vi "GIF.Read.Unpack__ogtk.vi"(6 "error in (no error)":errorcluster, 9 "Raw GIF89a bytes":u8[](array[numeric]) format="%.0x") -> (0 "error out":errorcluster, 2 "Delay (ms)":u32[](array[numeric]), 3 "Picture Array":T1[](array[typedef]))   [LabVIEW 2011]
uses:
  <vilib>/picture/picture.llb/imagedata.ctl
panel:
  out "Unpack in-progress":T2
  # "GIF.Read.Unpack.vi\n\nUnpacks image(s) from a raw GIF format.\n\nPlease visit http://www.OpenG.org to learn about the\nOpen Source LabVIEW software movement.\n\nNOTICE -- YOU MUST LEAVE THIS NOTICE IN PLACE.  PER THE TERMS OF THE LICENSE BELOW, YOU MAY SUBLICENSE THIS SOFTWARE \nIN ANY WAY THAT DOES NOT CONFLICT WITH THIS LICENSE.\n\n### BSD License (http://www.opensource.org/licenses/bsd-license.php) Begin ###\n \nCopyright (c) 2007, Bill Clench <bclench@yahoo.com>\n\nAll rights reserved.\n\nRedistribution and use in source and binary forms, with or without modification, are permitted provided that the following conditions are met:\n\n    * Redistributions of source code must retain the above copyright notice, this list of conditions and the following disclaimer.\n    * Redistributions in binary form must reproduce the above copyright notice, this list of conditions and the following disclaimer in the \n       documentation and/or other materials provided with the distribution.\n    * Neither the name of SciWare, James Kring, Inc., nor the names of its contributors may be used to endorse or promote products derived \n       from this software without specific prior written permission.\n\nTHIS SOFTWARE IS PROVIDED BY THE COPYRIGHT HOLDERS AND CONTRIBUTORS \"AS IS\" AND ANY EXPRESS OR IMPLIED WARRANTIES, \nINCLUDING, BUT NOT LIMITED TO, THE IMPLIED WARRANTIES OF MERCHANTABILITY AND FITNESS FOR A PARTICULAR PURPOSE ARE \nDISCLAIMED. IN NO EVENT SHALL THE COPYRIGHT OWNER OR CONTRIBUTORS BE LIABLE FOR ANY DIRECT, INDIRECT, INCIDENTAL,\n SPECIAL, EXEMPLARY, OR CONSEQUENTIAL DAMAGES (INCLUDING, BUT NOT LIMITED TO, PROCUREMENT OF SUBSTITUTE GOODS OR \nSERVICES; LOSS OF USE, DATA, OR PROFITS; OR BUSINESS INTERRUPTION) HOWEVER CAUSED AND ON ANY THEORY OF LIABILITY, \nWHETHER IN CONTRACT, STRICT LIABILITY, OR TORT (INCLUDING NEGLIGENCE OR OTHERWISE) ARISING IN ANY WAY OUT OF THE USE \nOF THIS SOFTWARE, EVEN IF ADVISED OF THE POSSIBILITY OF SUCH DAMAGE.\n\n### BSD License End ###"
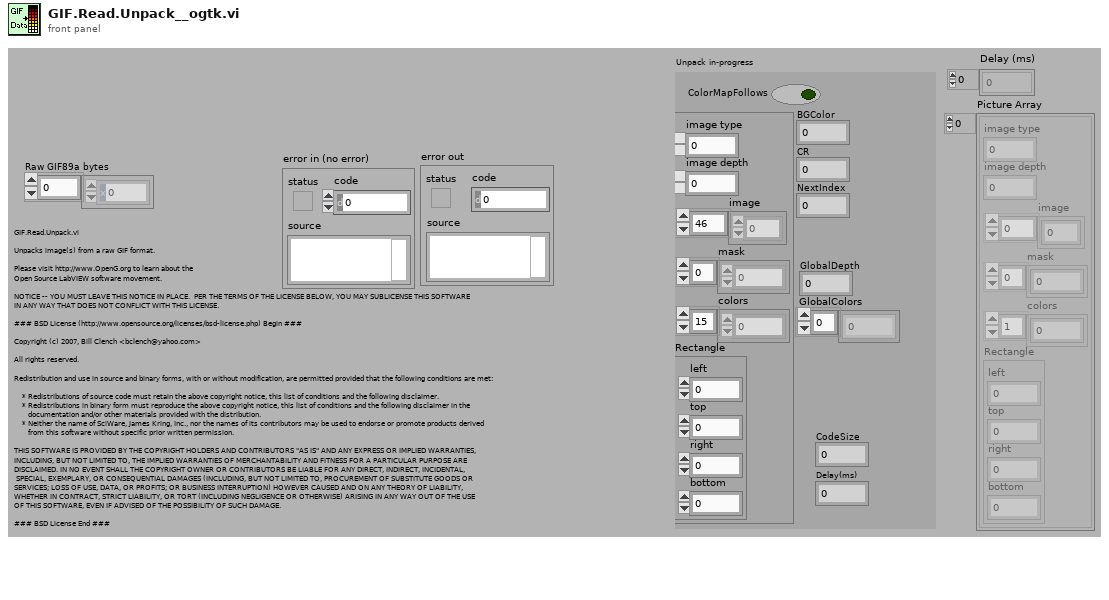
[diagram p1: front panel]
types:
  T1 = typedef "imagedata.ctl" = cluster{"image type":i32, "image depth":i32, "image":u8[], "mask":u8[], "colors":u32[], "Rectangle":cluster{"left":i16, "top":i16, "right":i16, "bottom":i16}}
  T2 = cluster{"ColorMapFollows":bool, "image data":T1, "BGColor":u8, "CR":u8, "NextIndex":i32, "GlobalDepth":i32, "CodeSize":i32, "Delay(ms)":i32, "GlobalColors":u32[]}
  T3 = enum16{"Begin", "Header", "LS_LSDescriptor", "LS_GCTable", "Data_LGD_SPB", "Data_GB_GRB_PTE", "Data_GB_GCE", "Data_GB_GRB_TBI_IDesc", "Data_GB_GRB_TBI_CMap", "Data_GB_GRB_TBI_ImageData", "End_Of_File"}
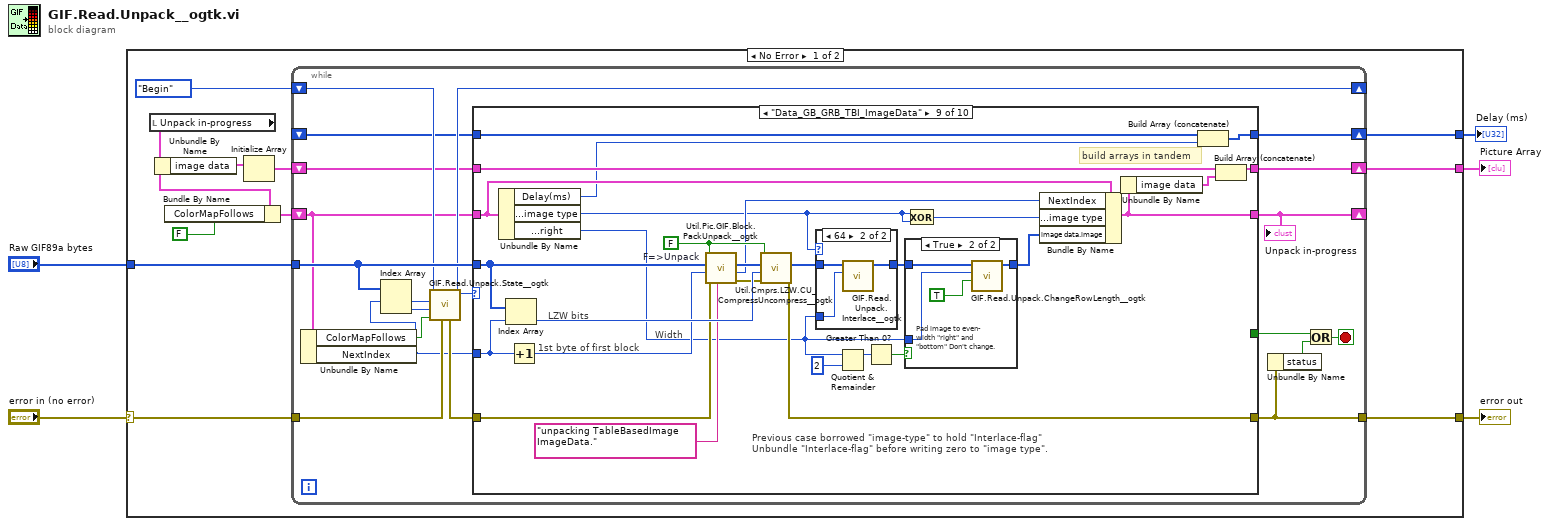
[diagram p0: block diagram]
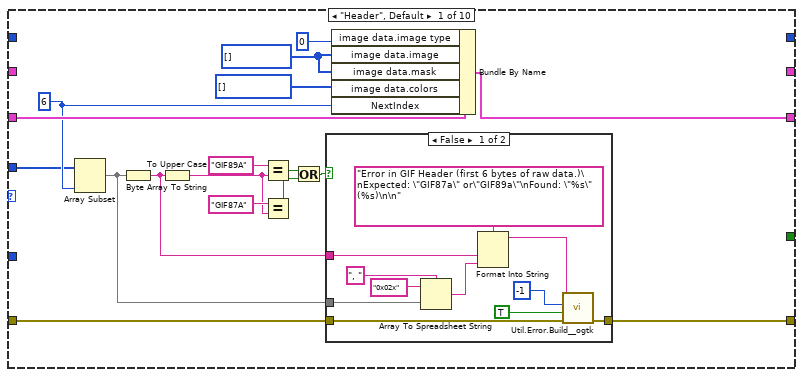
[diagram p2: hidden frame]
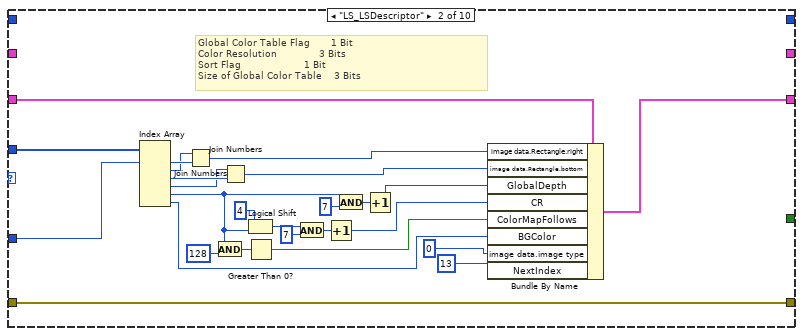
[diagram p4: hidden frame]
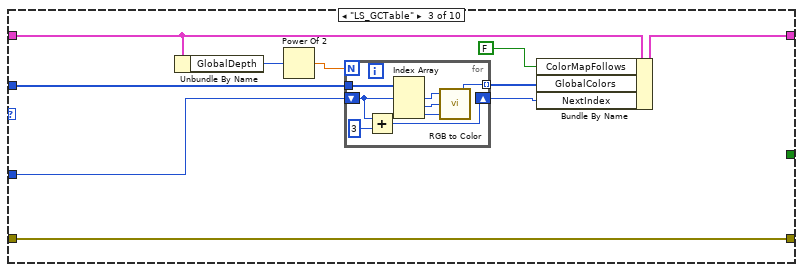
[diagram p5: hidden frame]
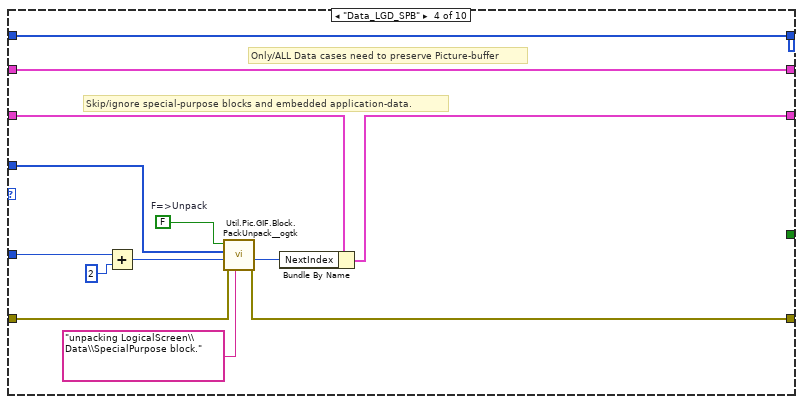
[diagram p6: hidden frame]
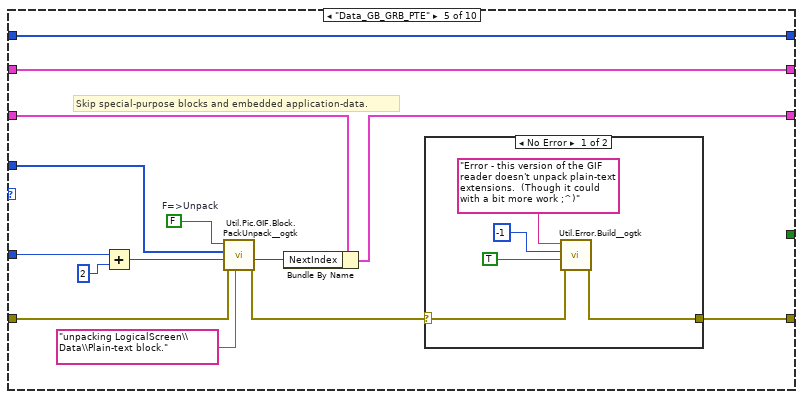
[diagram p7: hidden frame]
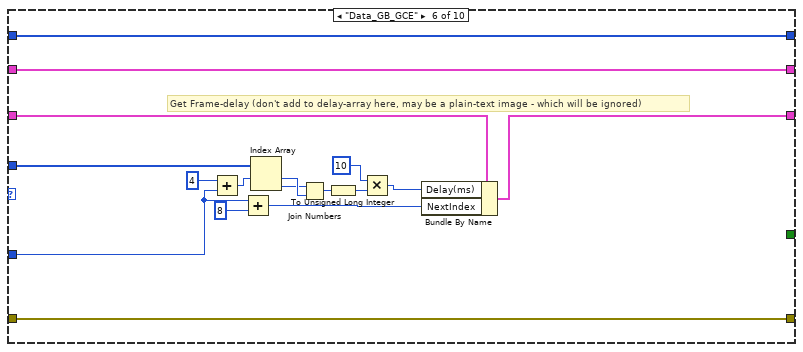
[diagram p9: hidden frame]
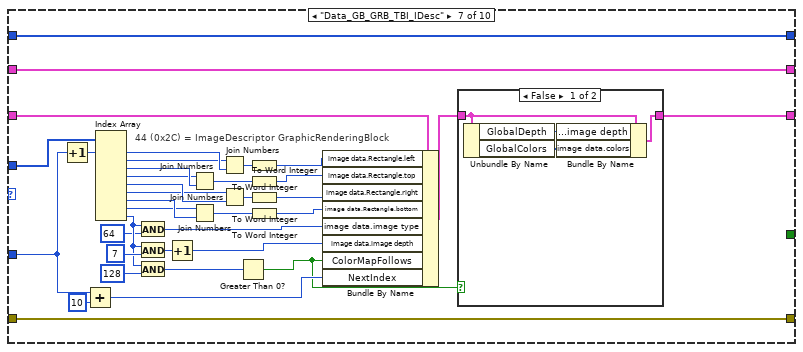
[diagram p10: hidden frame]
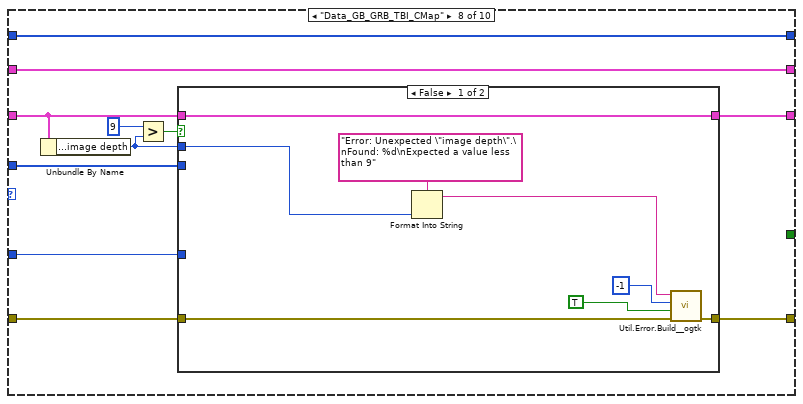
[diagram p12: hidden frame]
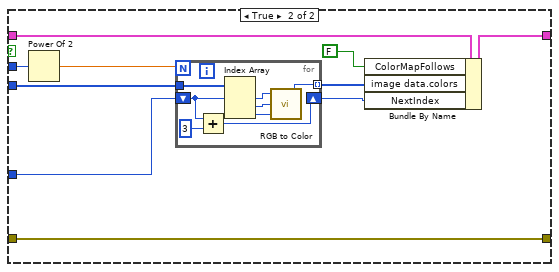
[diagram p13: hidden frame]
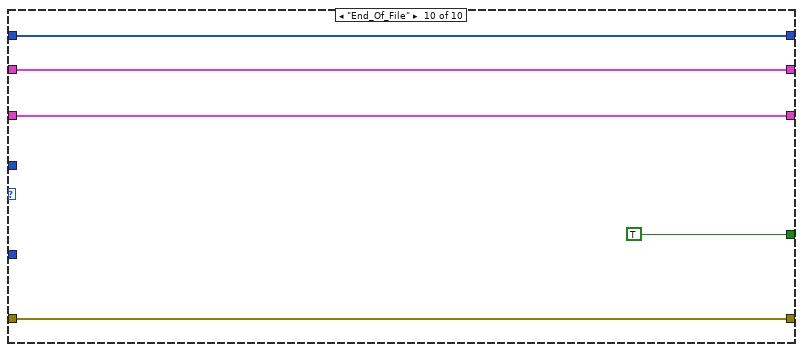
[diagram p16: hidden frame]
diagram:
  n1 = case shown="No Error" "error in (no error)" {
    selector: "error in (no error)" -> [w12 w279]
    tunnel: "Raw GIF89a bytes" -> [w16 _]
    tunnel: [w15 w279] -> w4
    tunnel: [w7 _] -> w2
    tunnel: [w6 _] -> w1
    frame No Error {
      n2 = local read "Unpack in-progress"() -> (w11:T2)
      n3 = Unbundle By Name(w11) -> ("image data"=w10:T1)
      n4 = Bundle By Name(cluster=w11, "ColorMapFollows"=FALSE) -> (w14:T2)
      n5 = Initialize Array(w10) -> (w9:T1[])  [unwired: 1 in]
      n6 = while {
        shift-right: [w28] -> _
        shift-left: w14 -> [w23]
        shift-right: [w26] -> _
        shift-left: T3."Begin" -> [w27]
        tunnel: w16 -> [w35]
        tunnel: [w32] -> w15
        tunnel: w12 -> [w25]
        shift-right: [w21] -> w7
        shift-left: w9 -> [w22]
        shift-right: [w18] -> w6
        shift-left: _ -> [w17]
        stop <- w30 stop-if-true
        n7 = Unbundle By Name(w23) -> ("ColorMapFollows"=w20:bool, "NextIndex"=w19:i32)
        n8 = Index Array(array=w35, index #1=w19) -> (element #1=w34:u8, element #2=w33:u8)  [unwired: 1 in]
        n9 = call "GIF.Read.Unpack.State__ogtk.vi"("error in (no error)"=w25, "ColorMap"=w20, "NextLabel"=w33, "NextCharacter"=w34, "State in"=w27) -> ("New State"=w26:T3, "error out"=w24:errorcluster)  [unwired: 5 in]
        n10 = case shown="\"Data_GB_GRB_TBI_ImageData\"" w26 {
          tunnel: w23 -> [w52 w68 w94 w120 w134 w150 w168 w208 w253 w278]
          tunnel: [w41 w65 w96 w119 w133 w149 w165 w207 w242 w278] -> w28
          tunnel: w35 -> [w40 w71 w98 w115 w129 w151 w171 w209 w260 _]
          tunnel: [w39 w66 w92 w112 w123 w147 w164 w201 w259 w276] -> w32
          tunnel: w19 -> [_ w67 w97 w118 w132 w148 w163 w210 w237 _]
          tunnel: [_ _ _ _ _ _ _ _ _ TRUE] -> w29
          tunnel: w24 -> [w37 w66 w92 w113 w126 w147 w164 w202 w249 w276]
          tunnel: w22 -> [_ _ _ w117 w131 w146 w170 w206 w257 w275]
          tunnel: [_ _ _ w117 w131 w146 w170 w206 w256 w275] -> w21
          tunnel: w17 -> [_ _ _ w109 w122 w142 w159 w200 w240 w274]
          tunnel: [_ _ _ w109 w122 w142 w159 w200 w239 w274] -> w18
          frame "Header", Default {
            w51 = u8[] []
            w42 = 6
            n11 = Array Subset(array=w40, length=w42) -> (w38:u8[])  [unwired: 1 in]
            n12 = Byte Array To String(unsigned byte array=w38) -> (string=w36:string)
            n13 = To Upper Case(1:w36) -> (0:w43:string)
            n14 = Equal?(x="GIF89A", y=w43) -> (x = y?=w47:bool)
            n15 = Equal?(x="GIF87A", y=w43) -> (x = y?=w46:bool)
            n16 = Or(x=w47, y=w46) -> (x .or. y?=w45:bool)
            n17 = case shown="False" w45 {
              tunnel: [w61 w64] -> w39
              tunnel: w36 -> [w62 _]
              tunnel: w38 -> [w57 _]
              tunnel: w37 -> [w53 w64]
              frame False {
                n18 = Array To Spreadsheet String(delimiter (Tab)=", ", array=w57, 3:"0x02x") -> (spreadsheet string=w54:string)
                n19 = Format Into String(format string="Error in GIF Header (first 6 bytes of raw data.)\nExpected: \"GIF87a\" or\"GIF89a\"\nFound: \"%s\" (%s)\n\n", w62, w54) -> (resulting string=w60:string)  [unwired: 2 in, 1 out]
                n20 = call "Util.Error.Build__ogtk.vi"("error in (no error)"=w53, "Status"=TRUE, "code"=-1, "Source"=w60) -> ("error out"=w61:errorcluster)  [unwired: 7 in]
              }
              frame True {
              }
            }
            n21 = Bundle By Name(cluster=w52, "image data.image type"=0, "image data.image"=w51, "image data.mask"=w51, "image data.colors"=u32[] [], "NextIndex"=w42) -> (w41:T2)
          }
          frame "LS_LSDescriptor" {
            # "Global Color Table Flag       1 Bit\nColor Resolution              3 Bits\nSort Flag                     1 Bit\nSize of Global Color Table    3 Bits"
            n22 = Index Array(array=w71, index #1=w67) -> (element #1=w90:u8, element #2=w89:u8, element #3=w88:u8, element #4=w87:u8, element #5=w77:u8, element #6=w79:u8)  [unwired: 5 in]
            n23 = Join Numbers(hi=w89, lo=w90) -> ((hi.lo)=w86:u16)
            n24 = And(x=w77, y=u8 128) -> (x .and. y?=w80:u8)
            n25 = Join Numbers(hi=w87, lo=w88) -> ((hi.lo)=w85:u16)
            n26 = Logical Shift(y=u8 4, x=w77) -> (x << y=w75:u8)
            n27 = Greater Than 0?(x=w80) -> (x > 0?=w72:bool)
            n28 = And(x=w75, y=u8 7) -> (x .and. y?=w74:u8)
            n29 = Increment(x=w74) -> (x+1=w73:u8)
            n30 = And(x=w77, y=u8 7) -> (x .and. y?=w82:u8)
            n31 = Increment(x=w82) -> (x+1=w81:u8)
            n32 = Bundle By Name(cluster=w68, "image data.Rectangle.right"=w86, "image data.Rectangle.bottom"=w85, "GlobalDepth"=w81, "CR"=w73, "ColorMapFollows"=w72, "BGColor"=w79, "image data.image type"=0, "NextIndex"=13) -> (w65:T2)
          }
          frame "LS_GCTable" {
            n33 = Unbundle By Name(w94) -> ("GlobalDepth"=w93:i32)
            n34 = Power Of 2(x=w93) -> (2^x=w100:dbl)
            n35 = for {
              N: w100 -> [_]
              shift-right: [w105] -> w99
              shift-left: w97 -> [w107]
              tunnel: w98 -> [w108]
              tunnel: [w101] -> w91 mode=indexing
              n36 = Add(x=w107, y=3) -> (x+y=w105:i32)
              n37 = Index Array(array=w108, index #1=w107) -> (element #1=w104:u8, element #2=w103:u8, element #3=w102:u8)  [unwired: 2 in]
              n38 = call <vilib>:"RGB to Color.vi"("B"=w102, "G"=w103, "R"=w104) -> ("Color"=w101:u32)
            }
            n39 = Bundle By Name(cluster=w94, "ColorMapFollows"=FALSE, "GlobalColors"=w91, "NextIndex"=w99) -> (w96:T2)
          }
          frame "Data_LGD_SPB" {
            w114 = FALSE  # F=>Unpack
            # "Only/ALL Data cases need to preserve Picture-buffer"
            # "Skip/ignore special-purpose blocks and embedded application-data."
            n40 = Add(x=w118, y=2 ("x")) -> (x+y=w116:i32)
            n41 = call "Util.Pic.GIF.Block.PackUnpack__ogtk.vi"("Calling routine"="unpacking LogicalScreen\\Data\\SpecialPurpose block.", "error in (no error)"=w113, "StartIndex"=w116, "BlockBytes in"=w115, "Pack/Unpack (T/F)"=w114) -> ("error out"=w112:errorcluster, "LastIndex"=w111:i32)  [unwired: 4 in, 1 out]
            n42 = Bundle By Name(cluster=w120, "NextIndex"=w111) -> (w119:T2)
          }
          frame "Data_GB_GRB_PTE" {
            w128 = FALSE  # F=>Unpack
            # "Skip special-purpose blocks and embedded application-data."
            n43 = Add(x=w132, y=2 ("x")) -> (x+y=w130:i32)
            n44 = call "Util.Pic.GIF.Block.PackUnpack__ogtk.vi"("Calling routine"="unpacking LogicalScreen\\Data\\Plain-text block.", "error in (no error)"=w126, "StartIndex"=w130, "BlockBytes in"=w129, "Pack/Unpack (T/F)"=w128) -> ("error out"=w125:errorcluster, "LastIndex"=w127:i32)  [unwired: 4 in, 1 out]
            n45 = Bundle By Name(cluster=w134, "NextIndex"=w127) -> (w133:T2)
            n46 = case shown="No Error" w125 {
              selector: w125 -> [w139 w141]
              tunnel: [w140 w141] -> w123
              frame No Error {
                n47 = call "Util.Error.Build__ogtk.vi"("error in (no error)"=w139, "Status"=TRUE, "code"=-1, "Source"="Error - this version of the GIF reader doesn't unpack plain-text extensions.  (Though it could with a bit more work ;^)") -> ("error out"=w140:errorcluster)  [unwired: 7 in]
              }
              frame Error {
              }
            }
          }
          frame "Data_GB_GCE" {
            # "Get Frame-delay (don't add to delay-array here, may be a plain-text image - which will be ignored)"
            n48 = Add(x=4, y=w148) -> (x+y=w154:i32)
            n49 = Add(x=w148, y=8 ("x")) -> (x+y=w152:i32)
            n50 = Index Array(array=w151, index #1=w154) -> (element #1=w157:u8, element #2=w156:u8)  [unwired: 1 in]
            n51 = Join Numbers(hi=w156, lo=w157) -> ((hi.lo)=w155:u16)
            n52 = To Unsigned Long Integer(number=w155) -> (unsigned 32bit integer=w145:u32)
            n53 = Multiply(x=u32 10, y=w145) -> (x*y=w143:u32)
            n54 = Bundle By Name(cluster=w150, "Delay(ms)"=w143, "NextIndex"=w152) -> (w149:T2)
          }
          frame "Data_GB_GRB_TBI_IDesc" {
            # "44 (0x2C) = ImageDescriptor GraphicRenderingBlock"
            n55 = Increment(x=w163) -> (x+1=w189:i32)
            n56 = Add(x=w163, y=10 ("x")) -> (x+y=w169:i32)
            n57 = Index Array(array=w171, index #1=w189) -> (element #1=w190:u8, element #2=w188:u8, element #3=w187:u8, element #4=w186:u8, element #5=w185:u8, element #6=w184:u8, element #7=w180:u8, element #8=w179:u8, element #9=w174:u8)  [unwired: 8 in]
            n58 = And(x=w174, y=u8 64) -> (x .and. y?=w172:u8)
            n59 = And(x=w174, y=u8 7) -> (x .and. y?=w175:u8)
            n60 = And(x=w174, y=u8 128) -> (x .and. y?=w192:u8)
            n61 = Increment(x=w175) -> (x+1=w160:u8)
            n62 = Join Numbers(hi=w186, lo=w187) -> ((hi.lo)=w182:u16)
            n63 = Join Numbers(hi=w179, lo=w180) -> ((hi.lo)=w194:u16)
            n64 = Join Numbers(hi=w188, lo=w190) -> ((hi.lo)=w183:u16)
            n65 = Join Numbers(hi=w184, lo=w185) -> ((hi.lo)=w181:u16)
            n66 = Greater Than 0?(x=w192) -> (x > 0?=w166:bool)
            n67 = To Word Integer(number=w183) -> (16bit integer=w177:i16)
            n68 = To Word Integer(number=w182) -> (16bit integer=w178:i16)
            n69 = To Word Integer(number=w181) -> (16bit integer=w162:i16)
            n70 = To Word Integer(number=w194) -> (16bit integer=w161:i16)
            n71 = Bundle By Name(cluster=w168, "image data.Rectangle.left"=w177, "image data.Rectangle.top"=w178, "image data.Rectangle.right"=w162, "image data.Rectangle.bottom"=w161, "image data.image type"=w172, "image data.image depth"=w160, "ColorMapFollows"=w166, "NextIndex"=w169) -> (w167:T2)
            n72 = case shown="False" w166 {
              tunnel: w167 -> [w197 w199]
              tunnel: [w198 w199] -> w165
              frame False {
                n73 = Unbundle By Name(w197) -> ("GlobalDepth"=w196:i32, "GlobalColors"=w195:u32[])
                n74 = Bundle By Name(cluster=w197, "image data.image depth"=w196, "image data.colors"=w195) -> (w198:T2)
              }
              frame True {
              }
            }
          }
          frame "Data_GB_GRB_TBI_CMap" {
            n75 = Unbundle By Name(w208) -> ("image data.image depth"=w204:i32)
            n76 = Greater?(x=9, y=w204) -> (0:w203:bool)
            n77 = case shown="False" w203 {
              tunnel: w210 -> [_ w226]
              tunnel: w209 -> [_ w225]
              tunnel: w208 -> [w218 w224]
              tunnel: [w218 w223] -> w207
              tunnel: w204 -> [w216 w220]
              tunnel: w202 -> [w214 w221]
              tunnel: [w215 w221] -> w201
              frame False {
                n78 = Format Into String(format string="Error: Unexpected \"image depth\".\nFound: %d\nExpected a value less than 9", w216) -> (resulting string=w213:string)  [unwired: 2 in, 1 out]
                n79 = call "Util.Error.Build__ogtk.vi"("error in (no error)"=w214, "Status"=TRUE, "code"=-1, "Source"=w213) -> ("error out"=w215:errorcluster)  [unwired: 7 in]
              }
              frame True {
                n80 = Power Of 2(x=w220) -> (2^x=w219:dbl)
                n81 = for {
                  N: w219 -> [_]
                  shift-right: [w233] -> w228
                  shift-left: w226 -> [w235]
                  tunnel: w225 -> [w236]
                  tunnel: [w229] -> w227 mode=indexing
                  n82 = Add(x=w235, y=3) -> (x+y=w233:i32)
                  n83 = Index Array(array=w236, index #1=w235) -> (element #1=w232:u8, element #2=w231:u8, element #3=w230:u8)  [unwired: 2 in]
                  n84 = call <vilib>:"RGB to Color.vi"("B"=w230, "G"=w231, "R"=w232) -> ("Color"=w229:u32)
                }
                n85 = Bundle By Name(cluster=w224, "ColorMapFollows"=FALSE, "image data.colors"=w227, "NextIndex"=w228) -> (w223:T2)
              }
            }
          }
          frame "Data_GB_GRB_TBI_ImageData" {
            w261 = FALSE  # F=>Unpack
            # "1st byte of first block"
            # "Width"
            # "build arrays in tandem"
            # "LZW bits"
            # "Previous case borrowed \"image-type\" to hold \"Interlace-flag\"\nUnbundle \"Interlace-flag\" before writing zero to \"image type\"."
            n86 = Unbundle By Name(w253) -> ("Delay(ms)"=w238:i32, "image data.image type"=w241:i32, "image data.Rectangle.right"=w245:i16)
            n87 = Index Array(array=w260, index=w237) -> (element=w264:u8)
            n88 = Increment(x=w237) -> (x+1=w263:i32)
            n89 = call "Util.Pic.GIF.Block.PackUnpack__ogtk.vi"("Calling routine"="unpacking TableBasedImage ImageData.", "error in (no error)"=w249, "StartIndex"=w263, "BlockBytes in"=w260, "Pack/Unpack (T/F)"=w261) -> ("error out"=w248:errorcluster, "LastIndex"=w244:i32, "BlockBytes out"=w262:u8[])  [unwired: 4 in]
            n90 = call "Util.Cmprs.LZW.CU_CompressUncompress__ogtk.vi"("error in (no error)"=w248, "LZWBits"=w264, "Data"=w262, "Compress/Decompress (T/F)"=w261) -> ("error out"=w259:errorcluster, "Data out"=w258:u8[])  [unwired: 6 in]
            n91 = case shown="64" w241 {
              tunnel: w258 -> [w270 w273]
              tunnel: [w270 w272] -> w250
              tunnel: w245 -> [_ w271]
              frame Default {
              }
              frame 64 {
                n92 = call "GIF.Read.Unpack.Interlace__ogtk.vi"("Columns"=w271, "Interlaced"=w273) -> ("Flat"=w272:u8[])  [unwired: 9 in]
              }
            }
            n93 = Quotient & Remainder(x=w245, y=i16 2) -> (x-y*floor(x/y)=w251:i16)  [unwired: 1 out]
            n94 = Greater Than 0?(x=w251) -> (x > 0?=w246:bool)
            n95 = case shown="True" w246 {
              tunnel: w250 -> [w265 w269]
              tunnel: w245 -> [_ w268]
              tunnel: [w265 w266] -> w243
              frame False {
              }
              frame True {
                # "Pad image to even-\nwidth \"right\" and\n\"bottom\" Don't change."
                n96 = call "GIF.Read.Unpack.ChangeRowLength__ogtk.vi"("+1/-1 (T/F)"=TRUE, "image width"=w268, "Image in"=w269) -> ("Image out"=w266:u8[])  [unwired: 8 in]
              }
            }
            n97 = Exclusive Or(1:w241, 2:w241) -> (0:w254:i32)
            n98 = Bundle By Name(cluster=w253, "NextIndex"=w244, "image data.image type"=w254, "image data.image"=w243) -> (w242:T2)
            n99 = Unbundle By Name(w242) -> ("image data"=w255:T1)
            n100 = Build Array (concatenate)(w240, w238) -> (w239:i32[])
            n101 = Build Array (concatenate)(w257, w255) -> (w256:T1[])
          }
          frame "End_Of_File" {
          }
        }
        "Unpack in-progress" <- w28
        n102 = Unbundle By Name(w32) -> ("status"=w31:bool)
        n103 = Or(x=w29, y=w31) -> (x .or. y?=w30:bool)
      }
    }
    frame Error {
    }
  }
  "error out" <- w4
  "Picture Array" <- w2
  "Delay (ms)" <- w1
